vi "wait.vi"(0 "HGF_Queue":refnum<class "HGF_Queue.lvclass">, 3 "msTimeout (-1)":i32=-1, 5 "error in (no error)":errorcluster, 9 "ignore previous (F)":bool) -> (14 "dup HGF_Queue":refnum<class "HGF_Queue.lvclass">, 16 "Object":refnum<class>, 17 "timed out":bool, 19 "error out":errorcluster)   [LabVIEW 2014, in "HGF_BaseClasses.lvlib" / "HGF_Queue.lvclass"]
doc: "Use this VI to wait for a Visitor for a time specified in timeout value. It returns the default object in case of timeout.\n\n<b>Hint:</b> This is a shared reentrant VI."
uses:
  HGF_Queue.lvclass
  HGF_Event/HGF_Event.lvclass
  HGF_Auxiliary/HGF_Auxiliary.lvlib
  HGF_Auxiliary/Severity.ctl
  HGF_Auxiliary/ErrorCode.ctl
  HGF_Timing/HGF_Timing.lvclass
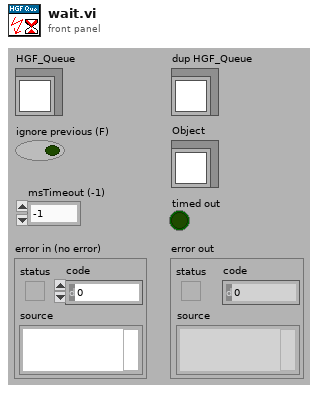
[diagram p1: front panel]
types:
  T1 = typedef "HGF_Auxiliary.lvlib/ErrorCode.ctl" = enum32{"No error", "Function not supported.", "This VI is for friends only.", "Reference object aready exisits.", "Parameter out of range.", "Not a rendezvous.", "Invalid notifier reference.", "Invalid queue reference.", "Self-Test not supported.", "Reset not supported.", "IDN query not supported.", "Error query not supported.", "Incorrect addressee.", "Object already exists.", "No class name specified", "Driver not supported", "Attribute is not writable"}
  T2 = typedef "HGF_Auxiliary.lvlib/Severity.ctl" = enum16{"Info", "Warning", "Fault", "Error", "Fatal"}
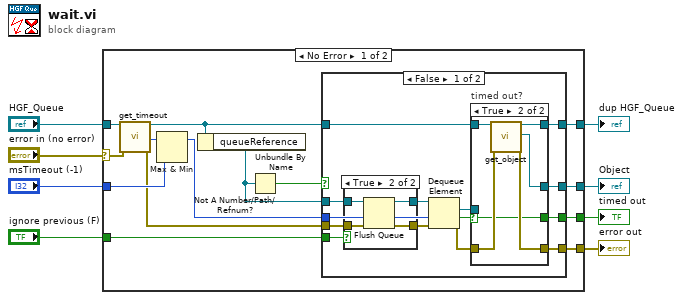
[diagram p0: block diagram]
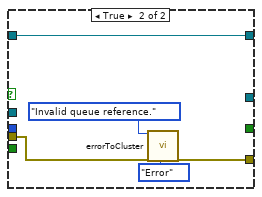
[diagram p4: hidden frame]
diagram:
  n1 = case shown="No Error" "error in (no error)" {
    selector: "error in (no error)" -> [w18 _]
    tunnel: "HGF_Queue" -> [w22 w58]
    tunnel: [w10 w58] -> w7
    tunnel: [w21 _] -> w6
    tunnel: [w20 _] -> w5
    tunnel: [w19 _] -> w4
    tunnel: "msTimeout (-1)" -> [w15 _]
    tunnel: "ignore previous (F)" -> [w13 _]
    frame No Error {
      n2 = call "get_timeout.vi"("HGF_Event.lvclass in"=w22, "error in (no error)"=w18) -> ("HGF_Event.lvclass out"=w9:refnum<class "HGF_Queue.lvclass">, "timeout"=w17:i32, "error out"=w14:errorcluster)  [unwired: 15 out]
      n3 = Max & Min(x=w17, y=w15) -> (max(x,y)=w16:i32)  [unwired: 1 out]
      n4 = Unbundle By Name(w9) -> ("queueReference"=w11:refnum<queue>)
      n5 = Not A Number/Path/Refnum?(number/path/refnum=w11) -> (NaN/Path/Refnum?=w12:bool)
      n6 = case shown="False" w12 {
        tunnel: [w27 _] -> w21
        tunnel: [w26 _] -> w20
        tunnel: [w23 w57] -> w19
        tunnel: w16 -> [w36 _]
        tunnel: w11 -> [w35 _]
        tunnel: w14 -> [w33 w55]
        tunnel: w13 -> [w31 _]
        tunnel: [w29 w53] -> w10
        tunnel: w9 -> [w30 w53]
        frame False {
          n7 = case shown="True" w31 {
            tunnel: w35 -> [w48 w52]
            tunnel: [w48 w51] -> w34
            tunnel: w33 -> [w47 w50]
            tunnel: [w47 w49] -> w32
            frame False {
            }
            frame True {
              n8 = Flush Queue(queue=w52, error in (no error)=w50) -> (queue out=w51:refnum<queue>, error out=w49:errorcluster)  [unwired: 1 out]
            }
          }
          n9 = Dequeue Element(queue=w34, timeout in ms (-1)=w36, error in (no error)=w32) -> (element=w25:refnum<class>, timed out?=w28:bool, error out=w24:errorcluster)  [unwired: 1 out]
          n10 = case "timed out?" shown="True" w28 {
            selector: w28 -> [w40 w42]
            tunnel: w30 -> [w38 w46]
            tunnel: [w38 w45] -> w29
            tunnel: w24 -> [w39 w44]
            tunnel: [w39 w43] -> w23
            tunnel: [w40 w42] -> w27
            tunnel: [w37 w41] -> w26
            tunnel: w25 -> [w37 _]
            frame False {
            }
            frame True {
              n11 = call "get_object.vi"("HGF_Timing.lvclass"=w46, "error in (no error)"=w44) -> ("dup HGF_Timing"=w45:refnum<class "HGF_Queue.lvclass">, "object"=w41:refnum<class>, "error out"=w43:errorcluster)  [unwired: 15 out]
            }
          }
        }
        frame True {
          n12 = call "errorToCluster.vi"("error code"=ErrorCode."Invalid queue reference.", "error in (no error)"=w55, "severity (Error)"=Severity."Error") -> ("error out"=w57:errorcluster)  [unwired: 2 in, 14 out]
        }
      }
    }
    frame Error {
    }
  }
  "error out" <- w4
  "dup HGF_Queue" <- w7
  "Object" <- w5
  "timed out" <- w6
